vi "Save Unguided Calibration.vi"(8 "error in (no error)":errorcluster, 10 "Channel (1)":i32=1, 11 "VISA resource name":refnum<visa-resource-name>) -> (0 "error out":errorcluster, 3 "VISA resource name out":refnum<visa-resource-name>)   [LabVIEW 2018, in "Keysight PNA Series.lvlib"]
doc: "Calculates the error terms using the selected method, and applies the error terms to the selected measurement, then saves the calibration error-terms to the channels Cal Register or a User Cal Set."
uses:
  Keysight PNA Series.lvlib
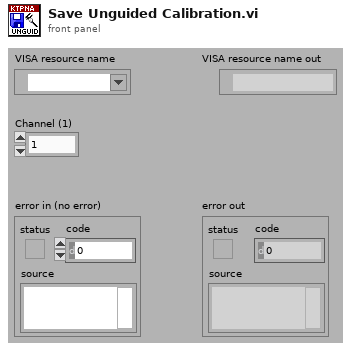
[diagram p1: front panel]
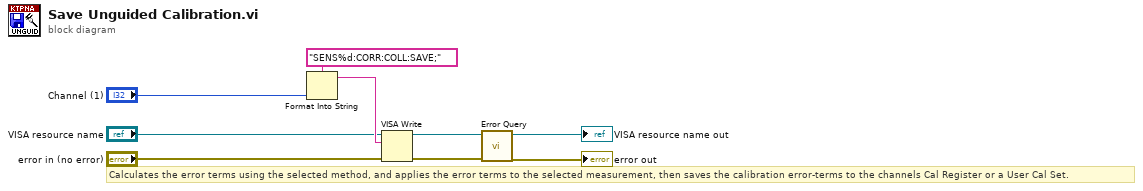
[diagram p0: block diagram]
diagram:
  # "Calculates the error terms using the selected method, and applies the error terms to the selected measurement, then saves the calibration error-terms to the channels Cal Register or a User Cal Set."
  n1 = Format Into String(format string="SENS%d:CORR:COLL:SAVE;", "Channel (1)") -> (resulting string=w7:string)  [unwired: 2 in, 1 out]
  n2 = VISA Write(VISA resource name="VISA resource name", write buffer=w7, error in (no error)="error in (no error)") -> (VISA resource name out=w4:refnum<visa-resource-name>, error out=w3:errorcluster)  [unwired: 1 out]
  n3 = call "Error Query.vi"("error in (no error)"=w3, "VISA resource name"=w4) -> ("error out"=→"error out":errorcluster, "VISA resource name out"=→"VISA resource name out":refnum<visa-resource-name>)  [unwired: 6 in, 2 out]
